vi "Subvi photon counter.vi"(5 "DI channel":refnum<k21>="Connector0/DIO1") -> (1 "PMT mon":bool, 2 "PMT edge change mon":bool, 3 "Gated pixel clock change mon":bool, 6 "Count":u8)   [LabVIEW 2017]
uses:
  <vilib>/rvi/eio/common/nirviEmuTemplateMethod_errors.vi
  GV gated pixel clock change.vi
  <vilib>/eio/EIONode/EIONode.xnode
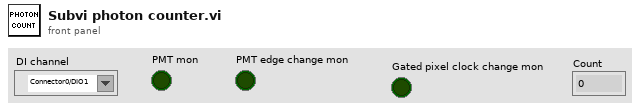
[diagram p1: front panel]
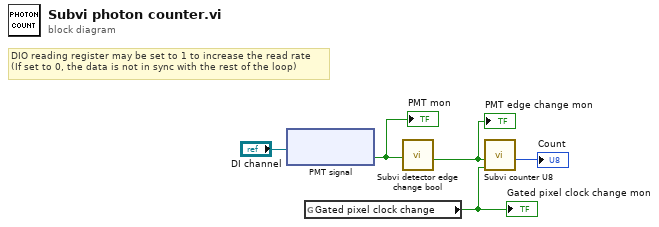
[diagram p0: block diagram]
diagram:
  # "DIO reading register may be set to 1 to increase the read rate\n(If set to 0, the data is not in sync with the rest of the loop)"
  n1 = xnode "PMT signal"("FPGA I/O In"="DI channel") -> ("I/O Item"=w4:bool)  [unwired: 1 out]
  "PMT mon" <- w4
  n2 = global read "GV gated pixel clock change.vi" "Gated pixel clock change"() -> (w2:bool)
  "Gated pixel clock change mon" <- w2
  n3 = call "Subvi detector edge change bool.vi"("Input"=w4) -> ("Output"=w3:bool)  [unwired: 8 in]
  "PMT edge change mon" <- w3
  n4 = call "Subvi counter U8.vi"("Reset"=w2, "+1"=w3) -> ("Count"=→"Count":u8)  [unwired: 9 in]
